vi "Find Time.vi"() -> (2 "Time":timestamp format="%<%x %.3X>T")   [LabVIEW 2020, in "jettl.lvlib"]
uses:
  jettl.lvlib
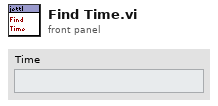
[diagram p1: front panel]
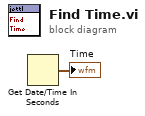
[diagram p0: block diagram]
diagram:
  n1 = Get Date/Time In Seconds() -> (seconds since 1Jan1904=→"Time":timestamp)
